vi "QCP_Close.vi"(11 "QCP_DevRef_In":T1) -> ()   [LabVIEW 2016]
uses:
  <userlib>/836-libraries/System/QCPv2/QCPSupportCode/QCP_RefNum.ctl
  <userlib>/836-libraries/System/QCPv2/QCPSupportCode/QCPData.ctl
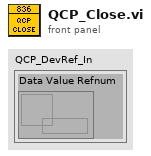
[diagram p1: front panel]
types:
  T1 = typedef "QCP_RefNum.ctl" = cluster{"Data Value Refnum":refnum<data-value>}
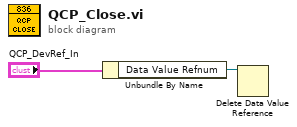
[diagram p0: block diagram]
diagram:
  n1 = Unbundle By Name("QCP_DevRef_In") -> ("Data Value Refnum"=w1:refnum<data-value>)
  n2 = Delete Data Value Reference(data value reference=w1) -> ()  [unwired: 1 in, 2 out]
